vi "check asynchronous errors.vi"(8 "error in":errorcluster, 11 "Module Info In":T1) -> (0 "error out":errorcluster, 2 "safe state?":bool, 3 "Module Info Out":T1)   [LabVIEW 2013, in "Standard Engine Runtime.lvclass"]
doc: "If an asynchronously running module returns an error, this VI checks the severity of the error as classified by that module and then executes the configured error actions. \n\nUnlike the synchronous version of this VI, execution decimation is not supported for Asynchronously running modules."
uses:
  Standard Engine Runtime.lvclass
  async execution info.ctl
  asynchronous process data.ctl
  async command notification.ctl
  <vilib>/NI/Tag Bus/table/data table.ctl
  <vilib>/NI/Tag Bus Module Framework/runtime/execution settings.ctl
  async error info.ctl
  <vilib>/NI/Tag Bus Module Framework/runtime/error classification.ctl
  Data Table with Transfer Spec.ctl
  <vilib>/NI/Tag Bus/table/transfer specification.ctl
  <vilib>/NI/Tag Bus/tag/Data Type.ctl
  Configuration/Module Decimation.ctl
  Configuration/Module Error Configuration.ctl
  Configuration/Error Actions By Category.ctl
  Configuration/Error Actions.ctl
  Configuration/Standard Engine Configuration.lvclass
  <vilib>/NI/Tag Bus Module Framework/runtime/TBM module execution interface.lvclass
  <vilib>/NI/Tag Bus/tag/tag descriptor.lvclass
  <vilib>/NI/Tag Bus/table/data table.lvlib
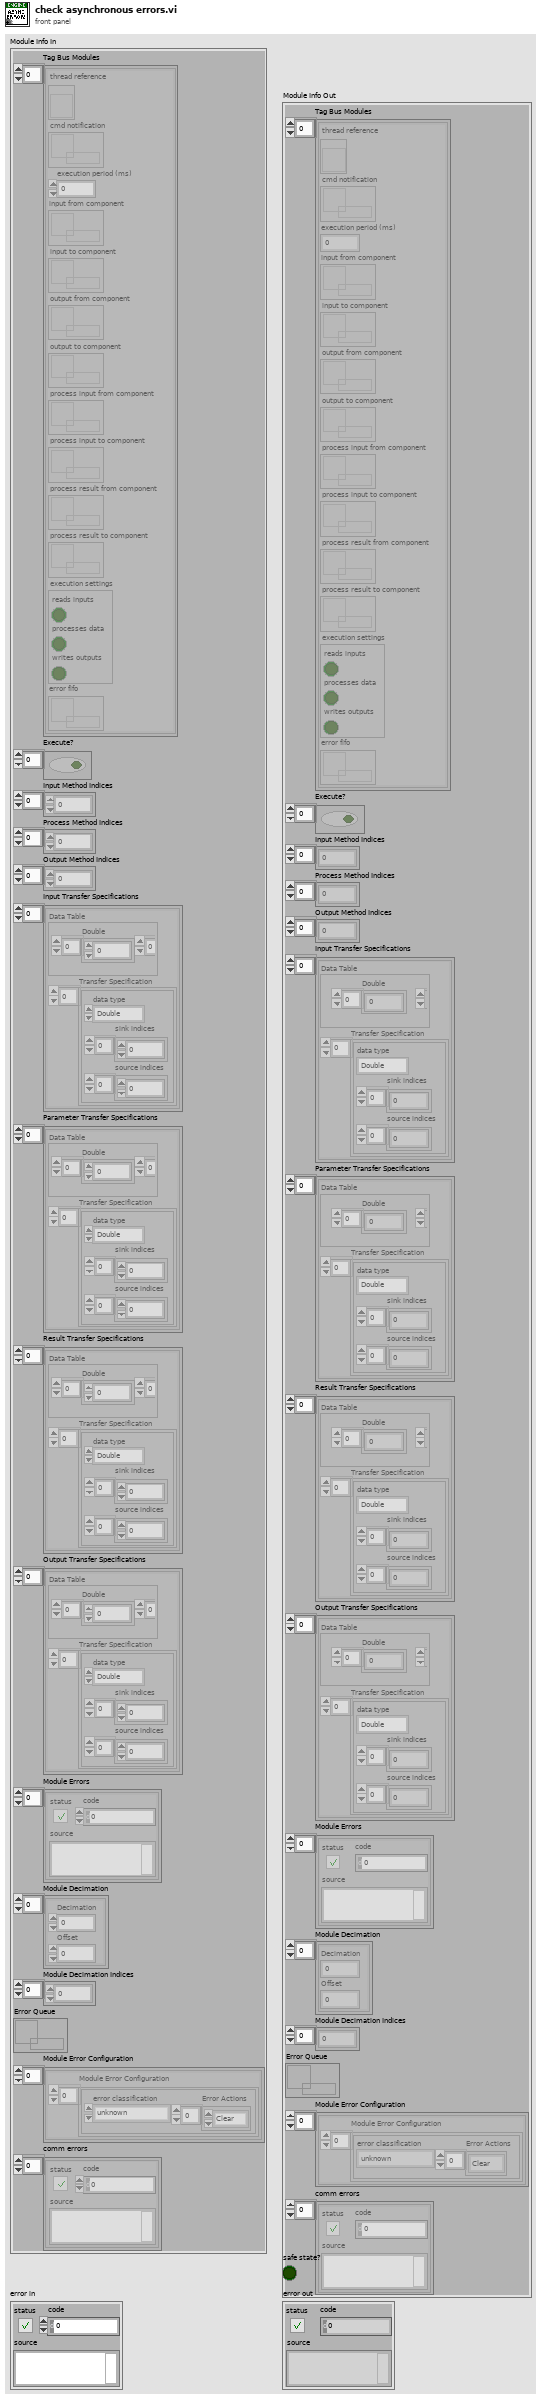
[diagram p1: front panel]
types:
  T1 = typedef "Standard Engine Runtime.lvclass/async execution info.ctl" = cluster{"Tag Bus Modules":T2[], "Execute?":bool[], "Input Method Indices":i32[], "Process Method Indices":i32[], "Output Method Indices":i32[], "Input Transfer Specifications":T4[], "Parameter Transfer Specifications":T4[], "Result Transfer Specifications":T4[], "Output Transfer Specifications":T4[], "Module Errors":errorcluster[], "Module Decimation":T8[], "Module Decimation Indices":i32[], "Error Queue":refnum<queue>, "Module Error Configuration":T9[], "comm errors":errorcluster[]}
  T2 = typedef "Standard Engine Runtime.lvclass/asynchronous process data.ctl" = cluster{"thread reference":refnum<vi>, "cmd notification":refnum<k33>, "execution period (ms)":i32, "input from component":refnum<queue>, "input to component":refnum<queue>, "output from component":refnum<queue>, "output to component":refnum<queue>, "process input from component":refnum<queue>, "process input to component":refnum<queue>, "process result from component":refnum<queue>, "process result to component":refnum<queue>, "execution settings":T3, "error fifo":refnum<k33>}
  T3 = typedef "TBM module execution interface.lvclass/execution settings.ctl" = cluster{"reads inputs":bool, "processes data":bool, "writes outputs":bool}
  T4 = typedef "Standard Engine Runtime.lvclass/Data Table with Transfer Spec.ctl" = cluster{"Data Table":T5, "Transfer Specification":T6[]}
  T5 = typedef "tag bus.lvlib/data table.lvlib/data table.ctl" = cluster{"Double":dbl[], "Single":sgl[], "I64":i64[], "I32":i32[], "I16":i16[], "I8":i8[], "U64":u64[], "U32":u32[], "U16":u16[], "U8":u8[], "Boolean":bool[], "String":string[], "Array of Double":cluster{"DBL Array":dbl[]}[], "Array of Single":cluster{"SGL Array":sgl[]}[], "Array of I64":cluster{"I64 Array":i64[]}[], "Array of I32":cluster{"I32 Array":i32[]}[], "Array of I16":cluster{"I16 Array":i16[]}[], "Array of I8":cluster{"I8 Array":i8[]}[], "Array of U64":cluster{"U64 Array":u64[]}[], "Array of U32":cluster{"U32 Array":u32[]}[], "Array of U16":cluster{"U16 Array":u16[]}[], "Array of U8":cluster{"U8 Array":u8[]}[], "Array of Boolean":cluster{"Boolean Array":bool[]}[], "Array of String":cluster{"String Array":string[]}[]}
  T6 = typedef "tag bus.lvlib/data table.lvlib/transfer specification.ctl" = cluster{"data type":T7, "sink indices":i32[], "source indices":i32[]}
  T7 = typedef "tag bus.lvlib/tag descriptor.lvclass/Data Type.ctl" = enum16{"Double", "Single", "I64", "I32", "I16", "I8", "U64", "U32", "U16", "U8", "Boolean", "String", "Array of Double", "Array of Single", "Array of I64", "Array of I32", "Array of I16", "Array of I8", "Array of U64", "Array of U32", "Array of U16", "Array of U8", "Array of Boolean", "Array of String"}
  T8 = typedef "Standard Engine Configuration.lvclass/Module Decimation.ctl" = cluster{"Decimation":u16, "Offset":u16}
  T9 = typedef "Standard Engine Configuration.lvclass/Module Error Configuration.ctl" = cluster{"Module Error Configuration":T10[]}
  T10 = typedef "Standard Engine Configuration.lvclass/Error Actions By Category.ctl" = cluster{"error classification":T11, "Error Actions":T12[]}
  T11 = typedef "TBM module execution interface.lvclass/error classification.ctl" = enum16{"unknown", "none", "trivial", "recoverable", "critical"}
  T12 = typedef "Standard Engine Configuration.lvclass/Error Actions.ctl" = enum16{"Clear", "Notify", "Stop Component", "Stop Engine", "Safe State", "Attempt Recovery"}
  T13 = typedef "Standard Engine Runtime.lvclass/async error info.ctl" = cluster{"error code":i32, "error classification":T11}
  T14 = typedef "Standard Engine Runtime.lvclass/async command notification.ctl" = enum16{"stop", "safe state", "recover", "clear error"}
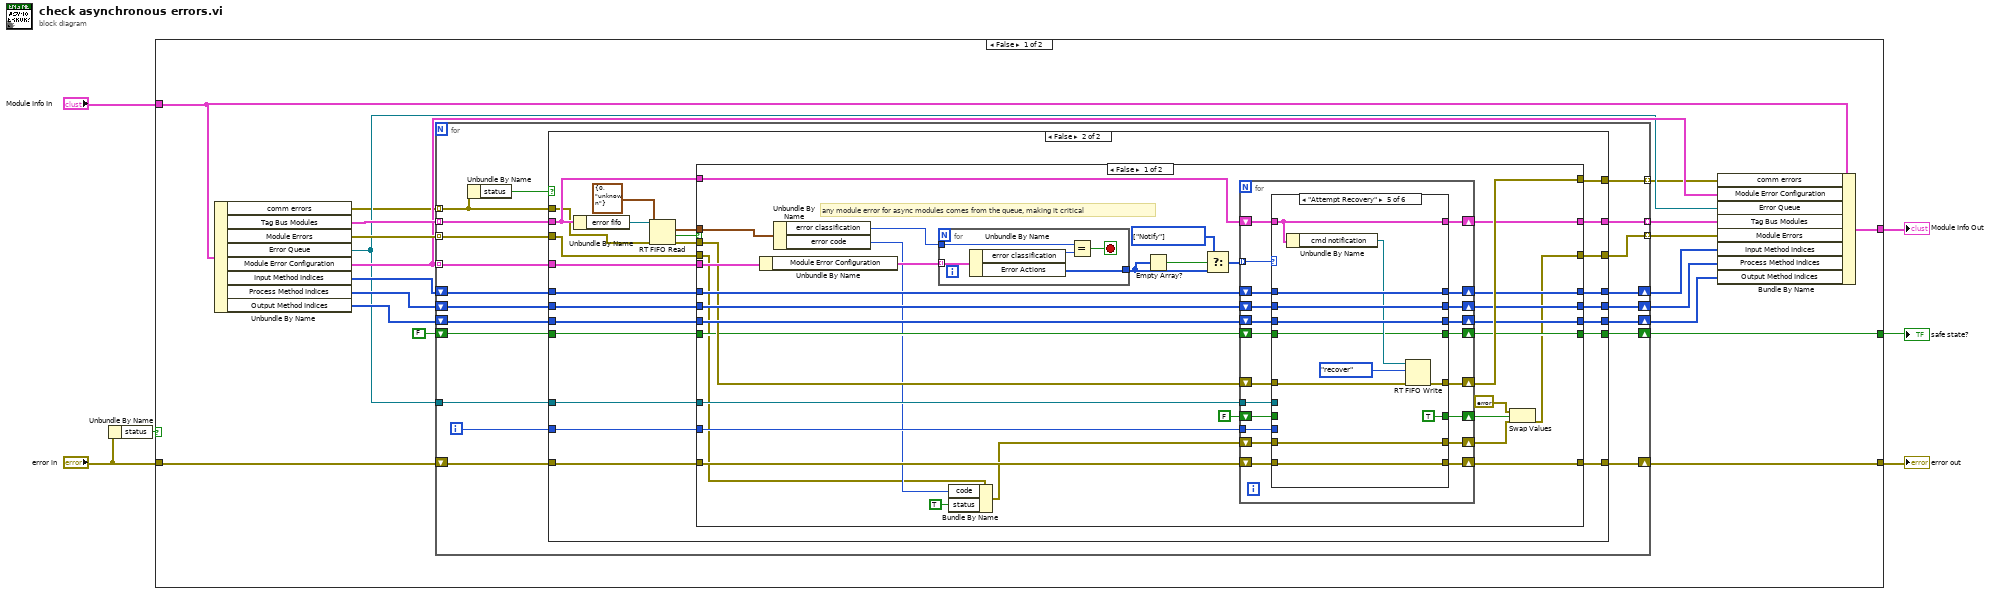
[diagram p0: block diagram]
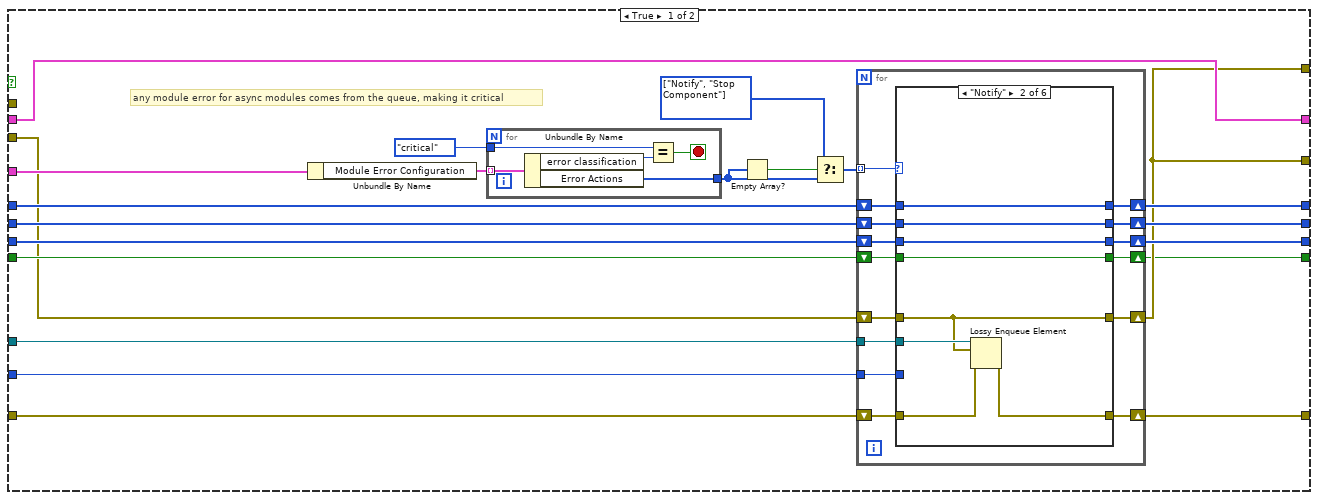
[diagram p2: hidden frame]
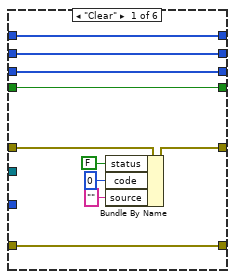
[diagram p3: hidden frame]
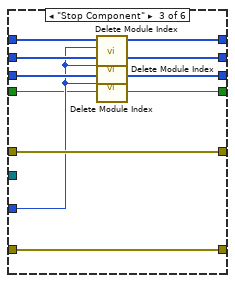
[diagram p4: hidden frame]
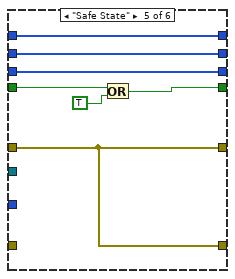
[diagram p6: hidden frame]
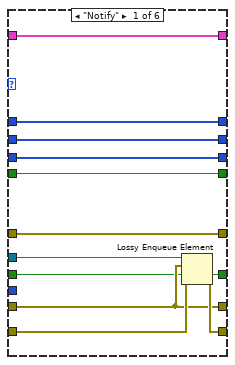
[diagram p8: hidden frame]
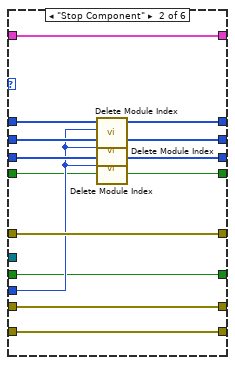
[diagram p9: hidden frame]
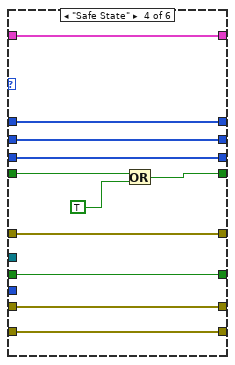
[diagram p11: hidden frame]
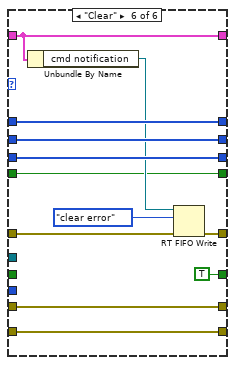
[diagram p12: hidden frame]
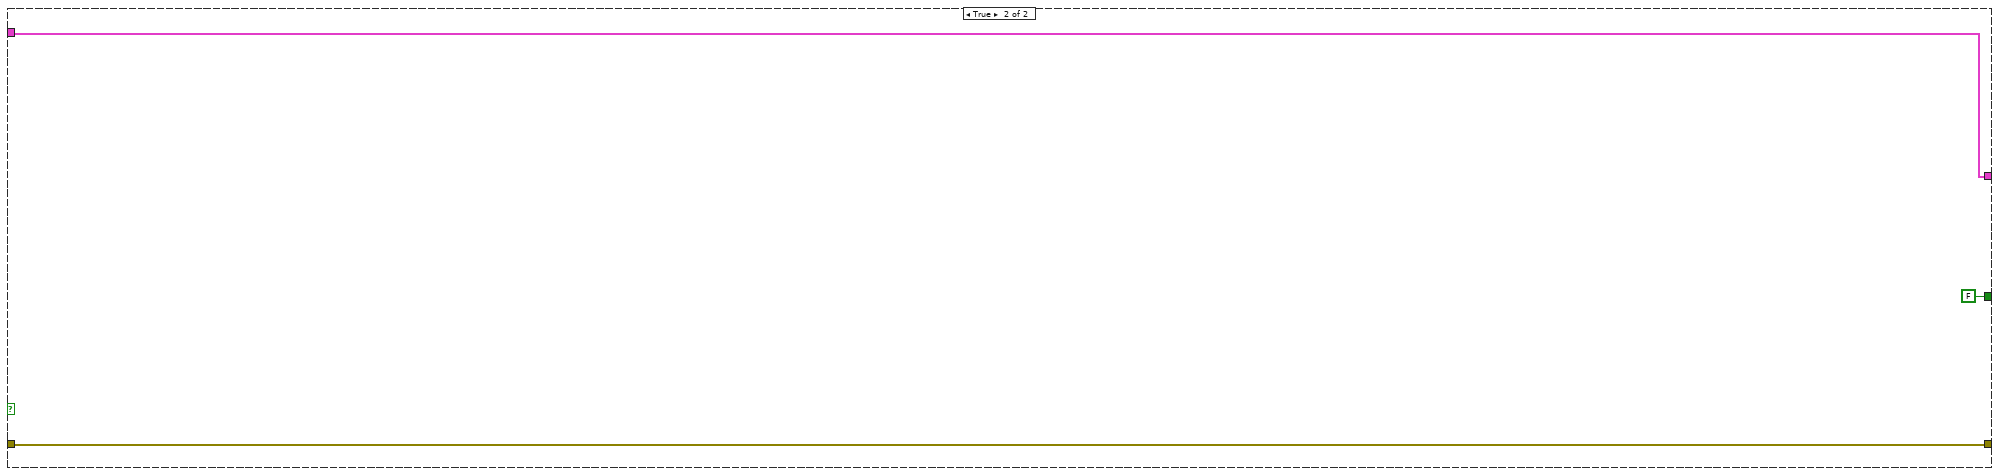
[diagram p14: hidden frame]
diagram:
  n1 = Unbundle By Name("error in") -> ("status"=w1:bool)
  n2 = case shown="False" w1 {
    tunnel: "Module Info In" -> [w16 w294]
    tunnel: "error in" -> [w15 w295]
    tunnel: [w14 w295] -> w5
    tunnel: [w13 w294] -> w4
    tunnel: [w9 FALSE] -> w3
    frame False {
      n3 = Unbundle By Name(w16) -> ("comm errors"=w8:errorcluster[], "Tag Bus Modules"=w26:T2[], "Module Errors"=w25:errorcluster[], "Error Queue"=w11:refnum<queue>, "Module Error Configuration"=w12:T9[], "Input Method Indices"=w22:i32[], "Process Method Indices"=w21:i32[], "Output Method Indices"=w20:i32[])
      n4 = for {
        tunnel: w25 -> [w30] mode=indexing
        tunnel: [w44] -> w23 mode=indexing
        tunnel: [w43] -> w24 mode=indexing
        tunnel: w26 -> [w41] mode=indexing
        tunnel: w12 -> [w42] mode=indexing
        shift-right: [w45] -> w14
        shift-left: w15 -> [w46]
        tunnel: w11 -> [w40]
        shift-right: [w36] -> w19
        shift-left: w22 -> [w39]
        shift-right: [w35] -> w18
        shift-left: w21 -> [w38]
        shift-right: [w34] -> w17
        shift-left: w20 -> [w37]
        shift-right: [w31] -> w9
        shift-left: FALSE -> [w32]
        tunnel: w8 -> [w27] mode=indexing
        tunnel: [w29] -> w7 mode=indexing
        i -> [w33]
        n5 = Unbundle By Name(w27) -> ("status"=w28:bool)
        n6 = case shown="False" w28 {
          tunnel: w46 -> [w68 w158]
          tunnel: [w67 w157] -> w45
          tunnel: [w50 w136] -> w44
          tunnel: [w52 w141] -> w43
          tunnel: w41 -> [w52 w142]
          tunnel: w42 -> [w58 w148]
          tunnel: w40 -> [w66 w156]
          tunnel: w39 -> [w65 w155]
          tunnel: w38 -> [w64 w154]
          tunnel: w37 -> [w63 w153]
          tunnel: [w62 w152] -> w36
          tunnel: [w61 w151] -> w35
          tunnel: [w60 w150] -> w34
          tunnel: w33 -> [w59 w149]
          tunnel: w32 -> [w49 w140]
          tunnel: [w48 w139] -> w31
          tunnel: w30 -> [w47 w137]
          tunnel: [w50 w138] -> w29
          tunnel: w27 -> [_ w135]
          frame True {
            w53 = T12[] [enum."Notify", enum."Stop Component"] items=["Clear", "Notify", "Stop Component", "Stop Engine", "Safe State", "Attempt Recovery"] ("t")
            # "any module error for async modules comes from the queue, making it critical"
            n7 = Unbundle By Name(w58) -> ("Module Error Configuration"=w57:T10[])
            n8 = for {
              tunnel: w57 -> [w73] mode=indexing
              tunnel: error_classification."critical" ("error classification") -> [w72]
              tunnel: [w69] -> w55
              stop <- w70 stop-if-true
              n9 = Unbundle By Name(w73) -> ("error classification"=w71:T11, "Error Actions"=w69:T12[])
              n10 = Equal?(x=w72, y=w71) -> (x = y?=w70:bool)
            }
            n11 = Empty Array?(array=w55) -> (empty?=w56:bool)
            n12 = Select(t=w53, s=w56, f=w55) -> (s? t:f=w54:T12[])
            n13 = for {
              tunnel: w54 -> [w88] mode=indexing
              shift-right: [w87] -> w50
              shift-left: w47 -> [w86]
              shift-right: [w84] -> w67
              shift-left: w68 -> [w85]
              tunnel: w66 -> [w83]
              shift-right: [w81] -> w62
              shift-left: w65 -> [w82]
              shift-right: [w79] -> w61
              shift-left: w64 -> [w80]
              shift-right: [w77] -> w60
              shift-left: w63 -> [w78]
              tunnel: w59 -> [w76]
              shift-right: [w75] -> w48
              shift-left: w49 -> [w74]
              n14 = case shown="\"Notify\"" w88 {
                tunnel: [w92 w100 w116 w121 w128 w134] -> w87
                tunnel: w86 -> [w98 w100 w116 w121 w128 w134]
                tunnel: w85 -> [w97 w101 w115 _ _ w133]
                tunnel: [w97 w105 w115 w121 w128 w133] -> w84
                tunnel: w83 -> [_ w106 _ _ _ _]
                tunnel: w82 -> [w96 w104 w114 w120 w127 w132]
                tunnel: [w96 w104 w113 w120 w127 w132] -> w81
                tunnel: w80 -> [w95 w103 w112 w119 w126 w131]
                tunnel: [w95 w103 w110 w119 w126 w131] -> w79
                tunnel: w78 -> [w94 w102 w111 w118 w125 w130]
                tunnel: [w94 w102 w109 w118 w125 w130] -> w77
                tunnel: w76 -> [_ _ w108 _ _ _]
                tunnel: [w93 w99 w107 w117 w123 w129] -> w75
                tunnel: w74 -> [w93 w99 w107 w117 w124 w129]
                frame "Clear" {
                  n15 = Bundle By Name(cluster=w98, "status"=FALSE, "code"=0, "source"="") -> (w92:errorcluster)
                }
                frame "Notify" {
                  n16 = Lossy Enqueue Element(queue=w106, element=w100, error in (no error)=w101) -> (error out=w105:errorcluster)  [unwired: 3 out]
                }
                frame "Stop Component" {
                  n17 = call "Delete Module Index.vi"("Index"=w108, "Module Indices"=w114) -> ("Module Indices"=w113:i32[])  [unwired: 9 in]
                  n18 = call "Delete Module Index.vi"("Index"=w108, "Module Indices"=w112) -> ("Module Indices"=w110:i32[])  [unwired: 9 in]
                  n19 = call "Delete Module Index.vi"("Index"=w108, "Module Indices"=w111) -> ("Module Indices"=w109:i32[])  [unwired: 9 in]
                }
                frame "Stop Engine" {
                  # "Passing an engine error out stops the engine."
                }
                frame "Safe State" {
                  n20 = Or(x=w124, y=TRUE ("Stop Engine")) -> (x .or. y?=w123:bool)
                }
                frame "Attempt Recovery" {
                }
              }
            }
          }
          frame False {
            n21 = Unbundle By Name(w142) -> ("error fifo"=w146:refnum<k33>)
            n22 = RT FIFO Read(0:w146, 1:T13 {"error code"=0, "error classification"=enum."unknown"} ("element"), 3:w135) -> (9:w143:T13, 10:w144:bool, 11:w147:errorcluster)  [unwired: 1 in, 2 out]
            n23 = case shown="False" w144 {
              tunnel: [w191 w291] -> w138
              tunnel: w158 -> [w190 w287]
              tunnel: [w189 w287] -> w157
              tunnel: w156 -> [w188 _]
              tunnel: w155 -> [w187 w290]
              tunnel: w154 -> [w186 w289]
              tunnel: w153 -> [w185 w288]
              tunnel: [w184 w290] -> w152
              tunnel: [w183 w289] -> w151
              tunnel: [w182 w288] -> w150
              tunnel: w149 -> [w181 _]
              tunnel: w148 -> [w180 _]
              tunnel: w147 -> [w174 w291]
              tunnel: w143 -> [w170 _]
              tunnel: w142 -> [w173 w292]
              tunnel: [w172 w292] -> w141
              tunnel: w140 -> [w169 w286]
              tunnel: [w168 w286] -> w139
              tunnel: w137 -> [w165 w285]
              tunnel: [w159 w285] -> w136
              frame False {
                w175 = T12[] [enum."Notify"] items=["Clear", "Notify", "Stop Component", "Stop Engine", "Safe State", "Attempt Recovery"] ("t")
                # "any module error for async modules comes from the queue, making it critical"
                n24 = Unbundle By Name(w180) -> ("Module Error Configuration"=w179:T10[])
                n25 = Unbundle By Name(w170) -> ("error classification"=w171:T11, "error code"=w166:i32)
                n26 = for {
                  tunnel: w179 -> [w196] mode=indexing
                  tunnel: w171 -> [w195]
                  tunnel: [w192] -> w177
                  stop <- w193 stop-if-true
                  n27 = Unbundle By Name(w196) -> ("error classification"=w194:T11, "Error Actions"=w192:T12[])
                  n28 = Equal?(x=w195, y=w194) -> (x = y?=w193:bool)
                }
                n29 = Bundle By Name(cluster=w165, "code"=w166, "status"=TRUE) -> (w164:errorcluster)
                n30 = Empty Array?(array=w177) -> (empty?=w178:bool)
                n31 = Select(t=w175, s=w178, f=w177) -> (s? t:f=w176:T12[])
                n32 = for {
                  tunnel: w176 -> [w217] mode=indexing
                  shift-right: [w216] -> w191
                  shift-left: w174 -> [w215]
                  shift-right: [w213] -> w189
                  shift-left: w190 -> [w214]
                  tunnel: w188 -> [w212]
                  shift-right: [w210] -> w184
                  shift-left: w187 -> [w211]
                  shift-right: [w208] -> w183
                  shift-left: w186 -> [w209]
                  shift-right: [w206] -> w182
                  shift-left: w185 -> [w207]
                  tunnel: w181 -> [w205]
                  shift-right: [w203] -> w172
                  shift-left: w173 -> [w204]
                  shift-right: [w202] -> w168
                  shift-left: w169 -> [w201]
                  shift-right: [w199] -> w160
                  shift-left: w164 -> [w200]
                  shift-right: [w197] -> w162
                  shift-left: FALSE -> [w198]
                  n33 = case shown="\"Attempt Recovery\"" w217 {
                    tunnel: [w222 w241 w249 w260 w266 w278] -> w216
                    tunnel: w215 -> [w222 w241 w249 w260 w272 w284]
                    tunnel: w214 -> [w223 w240 _ w255 w271 w283]
                    tunnel: [w227 w240 w243 w255 w271 w283] -> w213
                    tunnel: w212 -> [w228 _ _ _ _ _]
                    tunnel: w211 -> [w226 w239 w248 w259 w270 w282]
                    tunnel: [w226 w238 w248 w259 w270 w282] -> w210
                    tunnel: w209 -> [w225 w237 w247 w258 w269 w281]
                    tunnel: [w225 w235 w247 w258 w269 w281] -> w208
                    tunnel: w207 -> [w224 w236 w246 w257 w268 w280]
                    tunnel: [w224 w234 w246 w257 w268 w280] -> w206
                    tunnel: w205 -> [_ w233 _ _ _ _]
                    tunnel: w204 -> [w221 w232 w245 w256 w267 w279]
                    tunnel: [w221 w232 w245 w256 w267 w279] -> w203
                    tunnel: [w220 w231 w244 w253 w263 w275] -> w202
                    tunnel: w201 -> [w220 w231 w244 w254 w263 w275]
                    tunnel: w200 -> [w219 w230 w243 w251 w262 w274]
                    tunnel: [w219 w230 w243 w251 w262 w274] -> w199
                    tunnel: w198 -> [w218 w229 w242 w250 _ _]
                    tunnel: [w218 w229 w242 w250 TRUE TRUE] -> w197
                    frame "Notify" {
                      n34 = Lossy Enqueue Element(queue=w228, element=w219, error in (no error)=w223) -> (error out=w227:errorcluster)  [unwired: 3 out]
                    }
                    frame "Stop Component" {
                      n35 = call "Delete Module Index.vi"("Index"=w233, "Module Indices"=w239) -> ("Module Indices"=w238:i32[])  [unwired: 9 in]
                      n36 = call "Delete Module Index.vi"("Index"=w233, "Module Indices"=w237) -> ("Module Indices"=w235:i32[])  [unwired: 9 in]
                      n37 = call "Delete Module Index.vi"("Index"=w233, "Module Indices"=w236) -> ("Module Indices"=w234:i32[])  [unwired: 9 in]
                    }
                    frame "Stop Engine" {
                      # "Passing an engine error out stops the engine."
                    }
                    frame "Safe State" {
                      n38 = Or(x=w254, y=TRUE ("Stop Engine")) -> (x .or. y?=w253:bool)
                    }
                    frame "Attempt Recovery" {
                      n39 = Unbundle By Name(w267) -> ("cmd notification"=w265:refnum<k33>)
                      n40 = RT FIFO Write(0:w265, 1:async_command_notification."recover" ("notification"), 3:w272) -> (11:w266:errorcluster)  [unwired: 2 in, 3 out]
                    }
                    frame "Clear" {
                      n41 = Unbundle By Name(w279) -> ("cmd notification"=w277:refnum<k33>)
                      n42 = RT FIFO Write(0:w277, 1:async_command_notification."clear error" ("notification"), 3:w284) -> (11:w278:errorcluster)  [unwired: 2 in, 3 out]
                    }
                  }
                }
                n43 = Swap Values(12:errorcluster {"status"=FALSE, "code"=0, "source"=""} ("error out"), 13:w162, 14:w160) -> (3:w159:errorcluster)  [unwired: 1 out]
              }
              frame True {
              }
            }
          }
        }
      }
      n44 = Bundle By Name(cluster=w16, "comm errors"=w7, "Module Error Configuration"=w12, "Error Queue"=w11, "Tag Bus Modules"=w24, "Module Errors"=w23, "Input Method Indices"=w19, "Process Method Indices"=w18, "Output Method Indices"=w17) -> (w13:T1)
    }
    frame True {
    }
  }
  "Module Info Out" <- w4
  "error out" <- w5
  "safe state?" <- w3
